vi "CONNECT.vi"(8 "error in (no error)":errorcluster, 10 "PASSWORD":string="BoneDawg9192!", 11 "USER":string="ostep") -> (0 "error out":errorcluster, 2 "connection ref out":T1)   [LabVIEW 2018, in "MySQLTools.lvlib"]
uses:
  MySQLTools.lvlib
  <vilib>/addons/database/Connection.llb/Conn ObjectReference.ctl
  <vilib>/addons/database/Connection.llb/DB Tools Open Connec (Path).vi
  <vilib>/addons/database/NI_Database_API.lvlib
panel:
  out "UDL path out":path
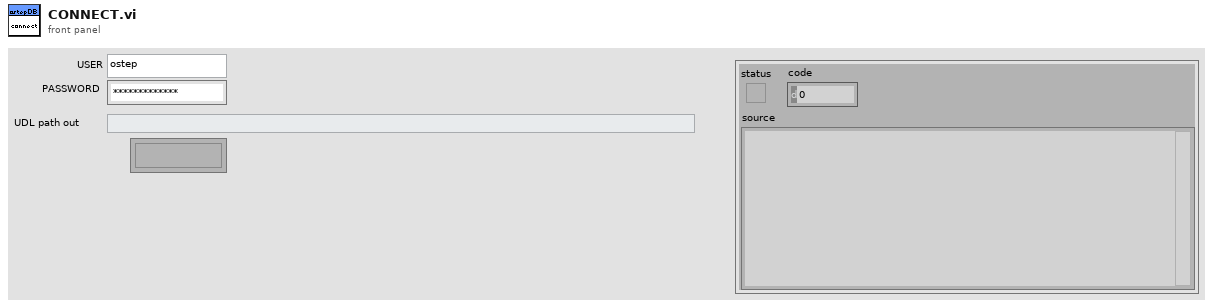
[diagram p1: front panel]
types:
  T1 = typedef "NI_Database_API.lvlib/Conn ObjectReference.ctl" = refnum<k1>
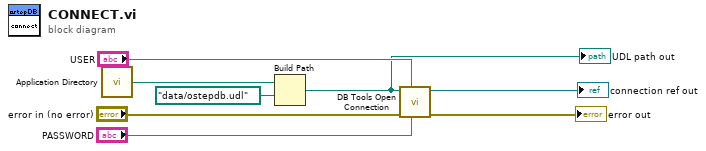
[diagram p0: block diagram]
diagram:
  n1 = call <vilib>:"Application Directory.vi"() -> ("Application Directory"=w3:path)
  n2 = Build Path(base path=w3, name or relative path=path "data/ostepdb.udl" ("connection information")) -> (appended path=w1:path)
  "UDL path out" <- w1
  n3 = call-poly <vilib>:"DB Tools Open Connection.vi"("password"="PASSWORD", "userID"="USER", "error in (no error)"="error in (no error)", "connection information"=w1) -> ("error out"=→"error out":errorcluster, "connection reference"=→"connection ref out":T1)  [unwired: 4 in]
